vi "Read Spartan Server Config.vi"(4 "error in (no error)":errorcluster, 7 "Config File Path (empty - use default)":path) -> (0 "error out":errorcluster, 3 "Config Keys":T1)   [LabVIEW 2011]
uses:
  ITK EXT/utils/keyedarr.llb/Keyed Array.ctl
  ITK EXT/utils/strutil.llb/Case Matching.ctl
  <vilib>/Utility/config.llb/Read Key (String).vi
  <vilib>/Utility/config.llb/NI_LVConfig.lvlib
panel:
  out "PROBE":cluster{"keys":string[], "values":string[]}
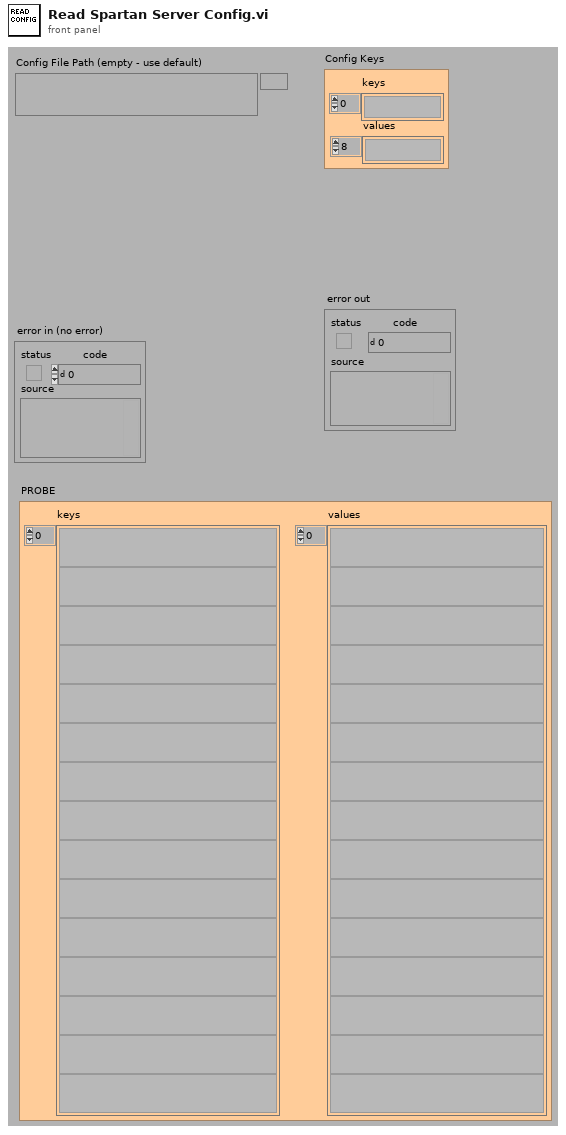
[diagram p1: front panel]
types:
  T1 = typedef "Keyed Array.ctl" = cluster{"keys":string[], "values":string[]}
  T2 = typedef "NI_LVConfig.lvlib/Config Data RefNum.ctl" = refnum<k1>
  T3 = typedef "Case Matching.ctl" = enum16{"a != A", "a == A", "system"}
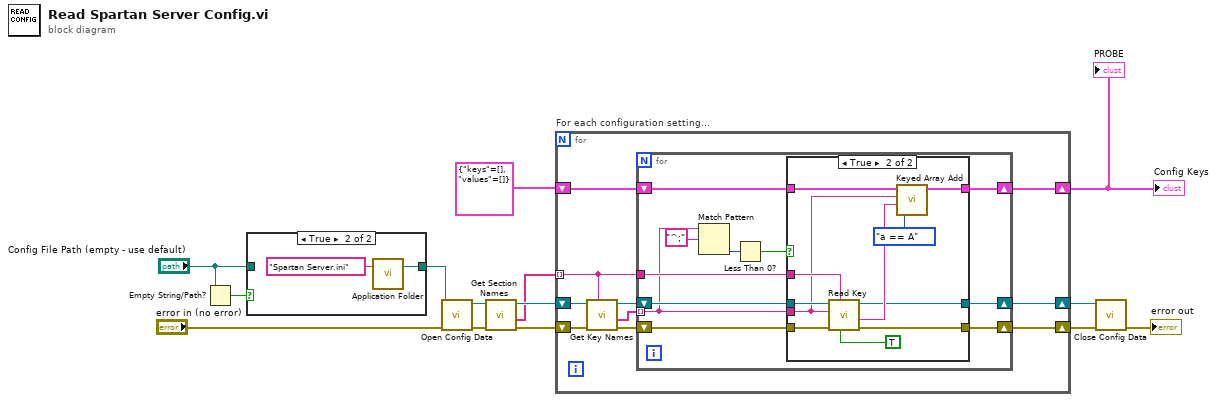
[diagram p0: block diagram]
diagram:
  n1 = Empty String/Path?(string/path="Config File Path (empty - use default)") -> (empty?=w8:bool)
  n2 = case shown="True" w8 {
    tunnel: [w15 w16] -> w9
    tunnel: "Config File Path (empty - use default)" -> [w15 _]
    frame False {
    }
    frame True {
      n3 = call "Application Folder.vi"("Relative Path (\"\" - Folder)"="Spartan Server.ini" ("regular expression")) -> ("Application Folder"=w16:path)  [unwired: 2 in]
    }
  }
  n4 = call <vilib>:"Open Config Data.vi"("error in (no error)"="error in (no error)", "configuration file path"=w9) -> ("error out"=w4:errorcluster, "refnum"=w6:T2)  [unwired: 7 in, 1 out]
  n5 = call <vilib>:"Get Section Names.vi"("error in (no error)"=w4, "refnum"=w6) -> ("error out"=w3:errorcluster, "section names"=w2:string[], "refnum out"=w5:T2)  [unwired: 7 in]
  n6 = for "For each configuration setting..." {
    shift-right: [w18] -> w13
    shift-left: w3 -> [w26]
    shift-right: [w19] -> w12
    shift-left: w5 -> [w27]
    shift-right: [w22] -> w1
    shift-left: T1 {"keys"=[], "values"=[]} ("array in") -> [w23]
    tunnel: w2 -> [w20] mode=indexing
    n7 = call <vilib>:"Get Key Names.vi"("section"=w20, "error in (no error)"=w26, "refnum"=w27) -> ("error out"=w24:errorcluster, "key names"=w21:string[], "refnum out"=w25:T2)  [unwired: 5 in, 1 out]
    n8 = for {
      shift-right: [w34] -> w19
      shift-left: w25 -> [w36]
      shift-right: [w33] -> w18
      shift-left: w24 -> [w35]
      shift-right: [w37] -> w22
      shift-left: w23 -> [w38]
      tunnel: w21 -> [w31] mode=indexing
      tunnel: w20 -> [w32]
      n9 = Match Pattern(string=w31, regular expression="^;") -> (offset past match=w29:i32)  [unwired: 1 in, 3 out]
      n10 = Less Than 0?(x=w29) -> (x < 0?=w28:bool)
      n11 = case shown="True" w28 {
        tunnel: w38 -> [w41 w51]
        tunnel: [w41 w50] -> w37
        tunnel: w36 -> [w40 w48]
        tunnel: w35 -> [w39 w47]
        tunnel: [w40 w46] -> w34
        tunnel: [w39 w45] -> w33
        tunnel: w32 -> [_ w44]
        tunnel: w31 -> [_ w43]
        frame False {
        }
        frame True {
          n12 = call-poly <vilib>:"Read Key.vi"("read raw string? (F)"=TRUE, "section"=w44, "error in (no error)"=w47, "key"=w43, "refnum"=w48) -> ("error out"=w45:errorcluster, "value"=w49:string, "refnum out"=w46:T2)  [unwired: 3 in, 1 out]
          n13 = call "Keyed Array Add.vi"("case matching (sensitive)"=Case_Matching."a == A", "value"=w49, "key"=w43, "array in"=w51) -> ("array out"=w50:T1)  [unwired: 3 out]
        }
      }
    }
  }
  "Config Keys" <- w1
  "PROBE" <- w1
  n14 = call <vilib>:"Close Config Data.vi"("error in (no error)"=w13, "refnum"=w12) -> ("error out"=→"error out":errorcluster)  [unwired: 1 in, 8 out]
